vi "PropPage_Decoration.vi"() -> (2 "OKtoQuit":bool)   [LabVIEW 2011]
doc: "Edit decorations position, size and foreground/background color.\n\n\nGeorge Zou\nhttp://webspace.webring.com/people/og/gtoolbox\n\n2016.6"
panel:
  in  "BGColor":u32(colorbox)=16777215 caption="BG Color"
  in  "FGColor":u32(colorbox) caption="FG Color"
  in  "Top":i32 caption="Top (pixel)" step=1
  in  "Left":i32 caption="Left (pixel)" step=1
  in  "Height":i32 caption="Height (pixel)" min=0 step=1
  in  "Width":i32 caption="Width (pixel)" min=0 step=1
  in  "idx":i32 caption="Index" min=0 step=1
  in  "all":bool caption="Apply to All ?"
  in  "QueueName":string
  in  "close":bool caption="Close"
  in  "Main Ref Array In":refnum<vi>[](array[refnum])
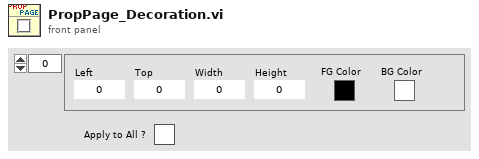
[diagram p1: front panel]
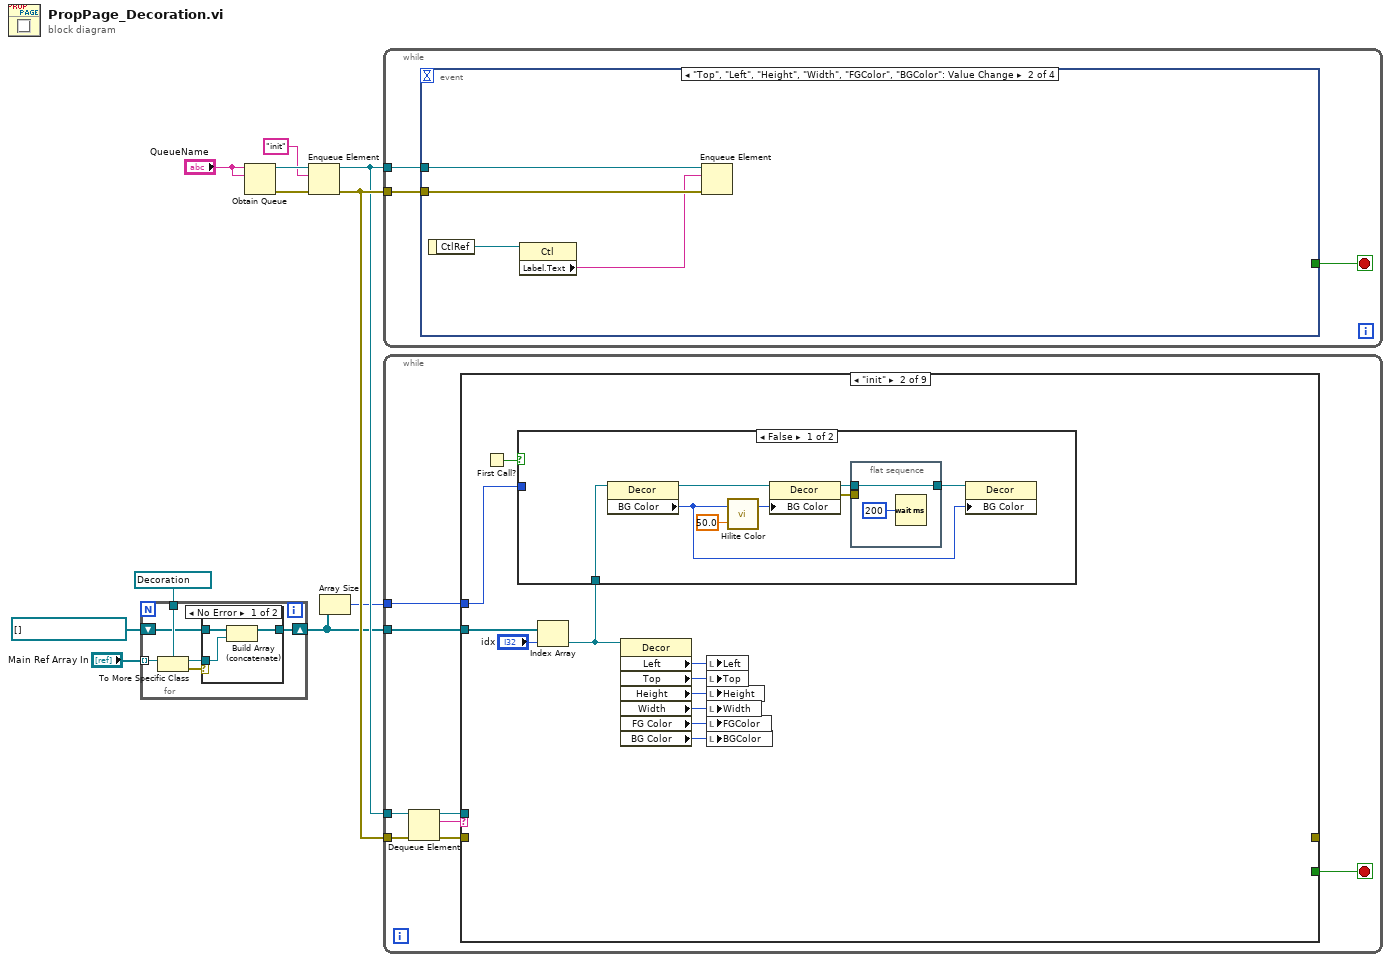
[diagram p0: block diagram]
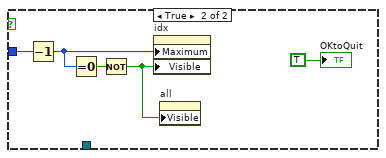
[diagram p4: hidden frame]
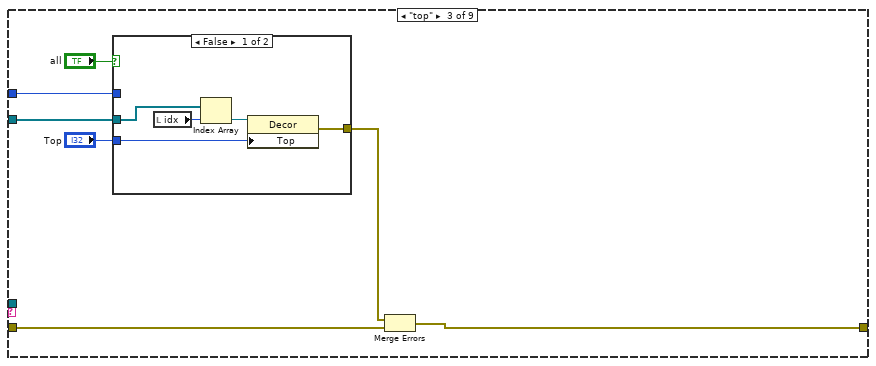
[diagram p5: hidden frame]
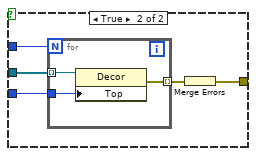
[diagram p6: hidden frame]
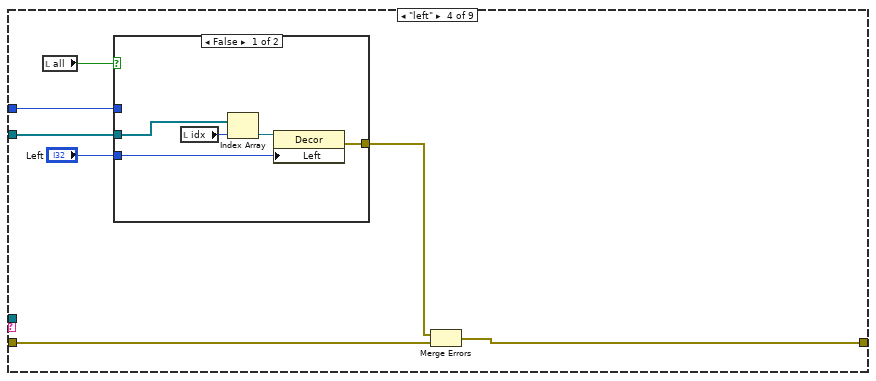
[diagram p7: hidden frame]
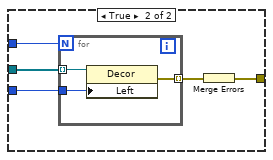
[diagram p8: hidden frame]
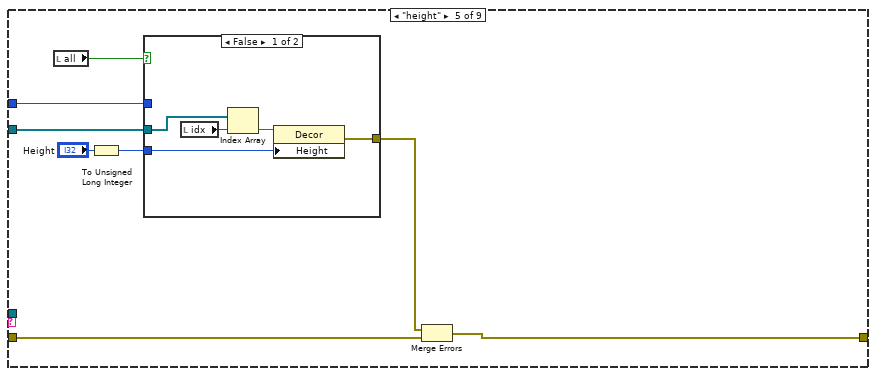
[diagram p9: hidden frame]
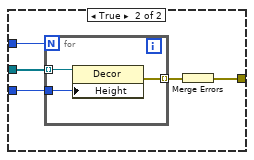
[diagram p10: hidden frame]
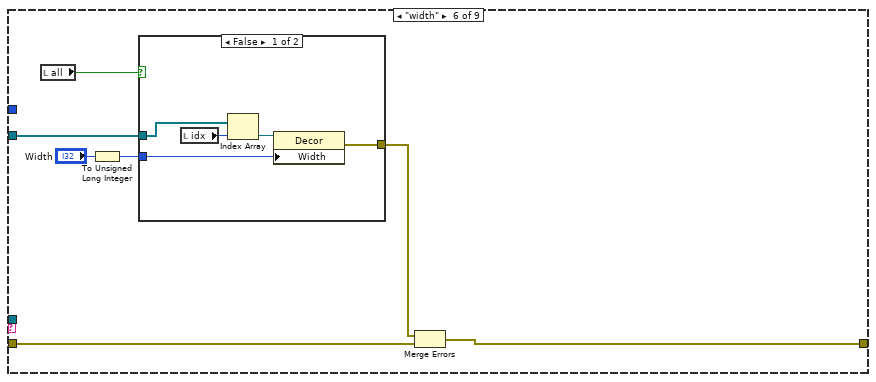
[diagram p11: hidden frame]
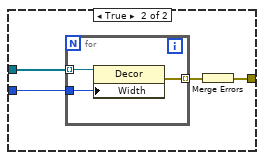
[diagram p12: hidden frame]
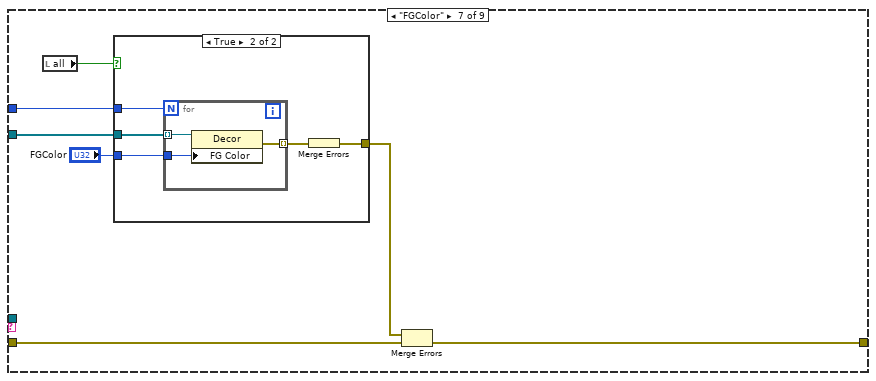
[diagram p13: hidden frame]
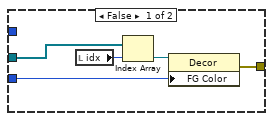
[diagram p14: hidden frame]
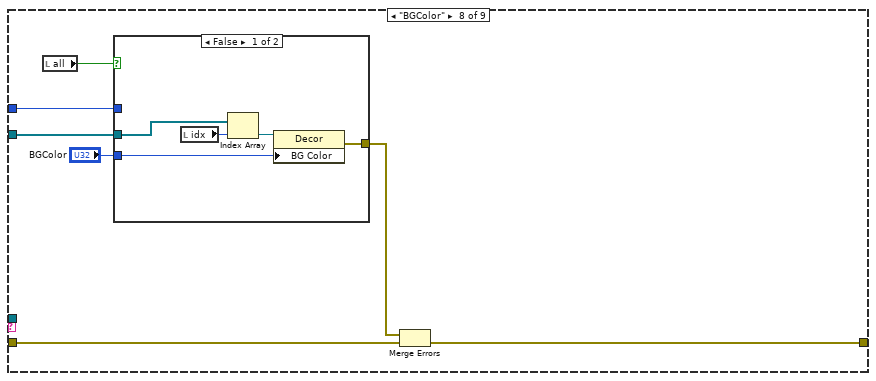
[diagram p15: hidden frame]
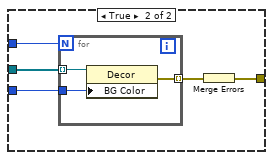
[diagram p16: hidden frame]
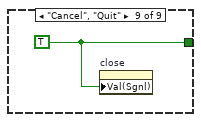
[diagram p17: hidden frame]
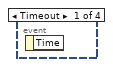
[diagram p18: hidden frame]
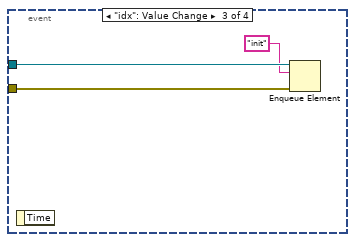
[diagram p19: hidden frame]
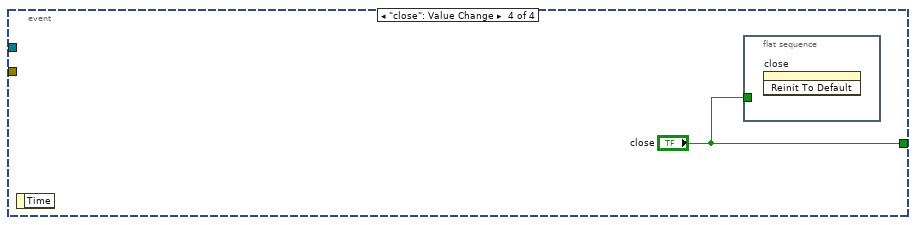
[diagram p20: hidden frame]
diagram:
  n1 = for {
    tunnel: "Main Ref Array In" -> [w17] mode=indexing
    tunnel: refnum<vi> refnum ("Decor Refnum") -> [w16]
    shift-right: [w13] -> w6
    shift-left: refnum<vi>[] [] -> [w14]
    n2 = To More Specific Class(target class=w16, reference=w17) -> (specific class reference=w12:refnum<vi>, error out=w15:errorcluster)  [unwired: 1 in]
    n3 = case shown="No Error" w15 {
      tunnel: w14 -> [w20 w21]
      tunnel: [w19 w21] -> w13
      tunnel: w12 -> [w18 _]
      frame No Error {
        n4 = Build Array (concatenate)(w20, w18) -> (w19:refnum<vi>[])
      }
      frame Error {
      }
    }
  }
  n5 = Obtain Queue(name (unnamed)="QueueName", element data type="QueueName") -> (queue out=w8:refnum<queue>, error out=w9:errorcluster)  [unwired: 3 in, 1 out]
  n6 = Enqueue Element(queue=w8, element="init" ("event"), error in (no error)=w9) -> (queue out=w7:refnum<queue>, error out=w10:errorcluster)  [unwired: 1 in, 1 out]
  n7 = Array Size(array=w6) -> (size(s)=w5:i32)
  n8 = while {
    tunnel: w7 -> [w24]
    tunnel: w10 -> [w23]
    stop <- w22 stop-if-true
    n9 = event shown="[1] \"Top\", \"Left\", \"Height\", \"Width\", \"FGColor\", \"BGColor\": Value Change" {
      selector: _ -> [_ _ _ _]
      dyn-events: _ -> [_ _ _ _]
      timeout: _ -> [_ _ _ _]
      tunnel: w24 -> [_ w28 w31 _]
      tunnel: w23 -> [_ w27 w30 _]
      tunnel: [_ _ _ "close"] -> w22
      event Timeout {
        n10 = event-data() -> ()  [unwired: 1 in, 1 out]
      }
      event "Top", "Left", "Height", "Width", "FGColor", "BGColor": Value Change {
        n11 = event-data() -> ("CtlRef"=w26:refnum<vi>)  [unwired: 1 in]
        n12 = property class="Ctl"(reference=w26) -> ("Label.Text"=w25:string)  [unwired: 1 in, 2 out]
        n13 = Enqueue Element(queue=w28, element=w25, error in (no error)=w27) -> ()  [unwired: 1 in, 3 out]
      }
      event "idx": Value Change {
        n14 = event-data() -> ()  [unwired: 1 in, 1 out]
        n15 = Enqueue Element(queue=w31, element="init" ("event"), error in (no error)=w30) -> ()  [unwired: 1 in, 3 out]
      }
      event "close": Value Change {
        n16 = event-data() -> ()  [unwired: 1 in, 1 out]
        n17 = flat-sequence {
          tunnel: "close" -> [_]
          frame #0 {
            n18 = invoke on="close" class="Bool (strict)" method="Reinit To Default"() -> ()  [unwired: 3 in, 3 out]
          }
        }
      }
    }
  }
  n19 = while {
    tunnel: w10 -> [w40]
    tunnel: w7 -> [w39]
    tunnel: w6 -> [w35]
    tunnel: w5 -> [w34]
    stop <- w37 stop-if-true
    n20 = Dequeue Element(queue=w39, error in (no error)=w40) -> (queue out=w36:refnum<queue>, element=w33:string, error out=w38:errorcluster)  [unwired: 1 in, 1 out]
    n21 = case shown="\"init\"" w33 {
      tunnel: w38 -> [_ _ w70 w90 w112 w132 w148 w168 _]
      tunnel: [_ _ _ _ _ _ _ _ w187] -> w37
      tunnel: w36 -> [_ _ _ _ _ _ _ _ _]
      tunnel: w35 -> [_ w51 w73 w93 w114 w134 w152 w172 _]
      tunnel: [_ _ w71 w91 w113 w133 w147 w167 _] -> _
      tunnel: w34 -> [_ w44 w67 w87 w107 _ w151 w171 _]
      frame Default {
      }
      frame "init" {
        n22 = First Call?() -> (First Call?: T/F=w45:bool)
        n23 = Index Array(array=w51, index="idx") -> (element=w41:refnum<vi>)
        n24 = case shown="False" w45 {
          tunnel: w44 -> [_ w66]
          tunnel: w41 -> [w59 _]
          frame False {
            n25 = property class="Decor"(reference=w59) -> (reference out=w58:refnum<vi>, "BG Color"=w53:u32)  [unwired: 1 in, 1 out]
            n26 = call <vilib>:"Hilite Color.vi"("Percentage(30)"=50.0, "Color In"=w53) -> ("Hilite"=w57:u32)  [unwired: 1 out]
            n27 = property class="Decor"(reference=w58, "BG Color"=w57) -> (reference out=w55:refnum<vi>, error out=w56:errorcluster)  [unwired: 1 in]
            n28 = flat-sequence {
              tunnel: w56 -> [_]
              tunnel: w55 -> [w60]
              tunnel: [w60] -> w54
              frame #0 {
                n29 = Wait (ms)(milliseconds to wait=u32 200) -> ()  [unwired: 1 out]
              }
            }
            n30 = property class="Decor"(reference=w54, "BG Color"=w53) -> ()  [unwired: 1 in, 2 out]
          }
          frame True {
            n31 = Decrement(x=w66) -> (x-1=w65:i32)
            n32 = Equal To 0?(x=w65) -> (x = 0?=w64:bool)
            n33 = Not(x=w64) -> (.not. x?=w62:bool)
            n34 = property on="idx" class="DigNum (strict)"("Maximum"=w65, "Visible"=w62) -> ()  [unwired: 2 in, 2 out]
            n35 = property on="all" class="Bool (strict)"("Visible"=w62) -> ()  [unwired: 2 in, 2 out]
            "OKtoQuit" <- TRUE ("OKtoQuit")
          }
        }
        n36 = property class="Decor"(reference=w41) -> ("Left"=w50:i32, "Top"=w49:i32, "Height"=w48:u32, "Width"=w47:u32, "FG Color"=w43:u32, "BG Color"=w42:u32)  [unwired: 1 in, 2 out]
        n37 = local write "Left"(w50) -> ()
        n38 = local write "Top"(w49) -> ()
        n39 = local write "Height"(w48) -> ()
        n40 = local write "Width"(w47) -> ()
        n41 = local write "FGColor"(w43) -> ()
        n42 = local write "BGColor"(w42) -> ()
      }
      frame "top" {
        n43 = case shown="False" "all" {
          tunnel: w73 -> [w78 w83]
          tunnel: [w74 w79] -> w72
          tunnel: "Top" -> [w75 w81]
          tunnel: w67 -> [_ w80]
          frame False {
            n44 = local read "idx"() -> (w77:i32)
            n45 = Index Array(array=w78, index=w77) -> (element=w76:refnum<vi>)
            n46 = property class="Decor"(reference=w76, "Top"=w75) -> (error out=w74:errorcluster)  [unwired: 1 in, 1 out]
          }
          frame True {
            n47 = for {
              N: w80 -> [_]
              tunnel: w83 -> [w86] mode=indexing
              tunnel: w81 -> [w85]
              tunnel: [w84] -> w82 mode=indexing
              n48 = property class="Decor"(reference=w86, "Top"=w85) -> (error out=w84:errorcluster)  [unwired: 1 in, 1 out]
            }
            n49 = Merge Errors(w82) -> (w79:errorcluster)
          }
        }
        n50 = Merge Errors(w72, w70) -> (w71:errorcluster)
      }
      frame "left" {
        n51 = local read "all"() -> (w88:bool)
        n52 = case shown="False" w88 {
          tunnel: w93 -> [w97 w103]
          tunnel: [w95 w99] -> w92
          tunnel: "Left" -> [w94 w101]
          tunnel: w87 -> [_ w100]
          frame False {
            n53 = local read "idx"() -> (w98:i32)
            n54 = Index Array(array=w97, index=w98) -> (element=w96:refnum<vi>)
            n55 = property class="Decor"(reference=w96, "Left"=w94) -> (error out=w95:errorcluster)  [unwired: 1 in, 1 out]
          }
          frame True {
            n56 = for {
              N: w100 -> [_]
              tunnel: w103 -> [w106] mode=indexing
              tunnel: w101 -> [w105]
              tunnel: [w104] -> w102 mode=indexing
              n57 = property class="Decor"(reference=w106, "Left"=w105) -> (error out=w104:errorcluster)  [unwired: 1 in, 1 out]
            }
            n58 = Merge Errors(w102) -> (w99:errorcluster)
          }
        }
        n59 = Merge Errors(w92, w90) -> (w91:errorcluster)
      }
      frame "height" {
        n60 = local read "all"() -> (w108:bool)
        n61 = To Unsigned Long Integer(number="Height") -> (unsigned 32bit integer=w111:u32)
        n62 = case shown="False" w108 {
          tunnel: w114 -> [w118 w124]
          tunnel: w111 -> [w117 w122]
          tunnel: [w115 w121] -> w109
          tunnel: w107 -> [_ w120]
          frame False {
            n63 = local read "idx"() -> (w119:i32)
            n64 = Index Array(array=w118, index=w119) -> (element=w116:refnum<vi>)
            n65 = property class="Decor"(reference=w116, "Height"=w117) -> (error out=w115:errorcluster)  [unwired: 1 in, 1 out]
          }
          frame True {
            n66 = for {
              N: w120 -> [_]
              tunnel: w124 -> [w127] mode=indexing
              tunnel: w122 -> [w126]
              tunnel: [w125] -> w123 mode=indexing
              n67 = property class="Decor"(reference=w127, "Height"=w126) -> (error out=w125:errorcluster)  [unwired: 1 in, 1 out]
            }
            n68 = Merge Errors(w123) -> (w121:errorcluster)
          }
        }
        n69 = Merge Errors(w109, w112) -> (w113:errorcluster)
      }
      frame "width" {
        n70 = local read "all"() -> (w128:bool)
        n71 = To Unsigned Long Integer(number="Width") -> (unsigned 32bit integer=w131:u32)
        n72 = case shown="False" w128 {
          tunnel: w134 -> [w138 w143]
          tunnel: w131 -> [w135 w141]
          tunnel: [w136 w140] -> w129
          frame False {
            n73 = local read "idx"() -> (w139:i32)
            n74 = Index Array(array=w138, index=w139) -> (element=w137:refnum<vi>)
            n75 = property class="Decor"(reference=w137, "Width"=w135) -> (error out=w136:errorcluster)  [unwired: 1 in, 1 out]
          }
          frame True {
            n76 = for {
              tunnel: w143 -> [w146] mode=indexing
              tunnel: w141 -> [w145]
              tunnel: [w144] -> w142 mode=indexing
              n77 = property class="Decor"(reference=w146, "Width"=w145) -> (error out=w144:errorcluster)  [unwired: 1 in, 1 out]
            }
            n78 = Merge Errors(w142) -> (w140:errorcluster)
          }
        }
        n79 = Merge Errors(w129, w132) -> (w133:errorcluster)
      }
      frame "FGColor" {
        n80 = local read "all"() -> (w153:bool)
        n81 = case shown="True" w153 {
          tunnel: w152 -> [w157 w163]
          tunnel: [w155 w159] -> w149
          tunnel: "FGColor" -> [w154 w161]
          tunnel: w151 -> [_ w160]
          frame False {
            n82 = local read "idx"() -> (w158:i32)
            n83 = Index Array(array=w157, index=w158) -> (element=w156:refnum<vi>)
            n84 = property class="Decor"(reference=w156, "FG Color"=w154) -> (error out=w155:errorcluster)  [unwired: 1 in, 1 out]
          }
          frame True {
            n85 = for {
              N: w160 -> [_]
              tunnel: w163 -> [w166] mode=indexing
              tunnel: w161 -> [w165]
              tunnel: [w164] -> w162 mode=indexing
              n86 = property class="Decor"(reference=w166, "FG Color"=w165) -> (error out=w164:errorcluster)  [unwired: 1 in, 1 out]
            }
            n87 = Merge Errors(w162) -> (w159:errorcluster)
          }
        }
        n88 = Merge Errors(w149, w148) -> (w147:errorcluster)
      }
      frame "BGColor" {
        n89 = local read "all"() -> (w173:bool)
        n90 = case shown="False" w173 {
          tunnel: w172 -> [w177 w183]
          tunnel: [w175 w179] -> w169
          tunnel: "BGColor" -> [w174 w181]
          tunnel: w171 -> [_ w180]
          frame False {
            n91 = local read "idx"() -> (w178:i32)
            n92 = Index Array(array=w177, index=w178) -> (element=w176:refnum<vi>)
            n93 = property class="Decor"(reference=w176, "BG Color"=w174) -> (error out=w175:errorcluster)  [unwired: 1 in, 1 out]
          }
          frame True {
            n94 = for {
              N: w180 -> [_]
              tunnel: w183 -> [w186] mode=indexing
              tunnel: w181 -> [w185]
              tunnel: [w184] -> w182 mode=indexing
              n95 = property class="Decor"(reference=w186, "BG Color"=w185) -> (error out=w184:errorcluster)  [unwired: 1 in, 1 out]
            }
            n96 = Merge Errors(w182) -> (w179:errorcluster)
          }
        }
        n97 = Merge Errors(w169, w168) -> (w167:errorcluster)
      }
      frame "Cancel", "Quit" {
        w187 = TRUE
        n98 = property on="close" class="Bool (strict)"("Val(Sgnl)"=w187) -> ()  [unwired: 2 in, 2 out]
      }
    }
  }
